vi "MTM2_monitorCommand_resetForceOffsets.vi"(8 "error in (no error)":errorcluster, 11 "command_resetForceOffsets_Ctl":T1) -> (0 "error out":errorcluster, 2 "function return":i32, 3 "command_resetForceOffsets_Ctl out":T1)   [LabVIEW 2018, in "SALLV_MTM2.lvlib"]
doc: "int MTM2_shm_monitorCommand_resetForceOffsetsLV(MTM2_command_resetForceOffsetsLV *command_resetForceOffsets_Ctl );"
uses:
  DataTypes/command_resetForceOffsets.ctl
  SALLV_MTM2.lvlib
  SALLV_MTM2.so
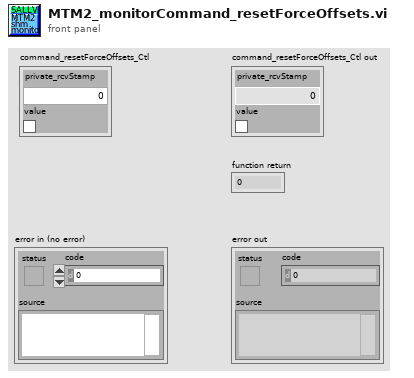
[diagram p1: front panel]
types:
  T1 = typedef "SALLV_MTM2.lvlib/command_resetForceOffsets.ctl" = cluster{"private_rcvStamp":dbl, "value":bool}
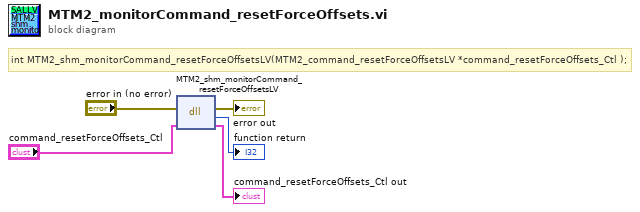
[diagram p0: block diagram]
diagram:
  # "int MTM2_shm_monitorCommand_resetForceOffsetsLV(MTM2_command_resetForceOffsetsLV *command_resetForceOffsets_Ctl );"
  n1 = dll-call lib="home/ttsai/Documents/salLabviewApi/SALLV_MTM2/SALLV_MTM2.*" fn="MTM2_shm_monitorCommand_resetForceOffsetsLV"(error in="error in (no error)", "command_resetForceOffsets_Ctl"="command_resetForceOffsets_Ctl") -> (error out=→"error out":errorcluster, →"function return":i32, "command_resetForceOffsets_Ctl"=→"command_resetForceOffsets_Ctl out":T1)  [unwired: 2 in, 1 out]
